vi "example-VariantArrayAccess.vi"() -> ()   [LabVIEW 2020]
uses:
  VariantArrayAccessMulti.vi
panel:
  in  "New Value":cxt
  out "Old Value":variant
  out "Revised Array":variant
  in  "Numeric Array as Variant 2":variant
  out "element":variant
  in  "index":i32
  in  "Array as Variant":variant
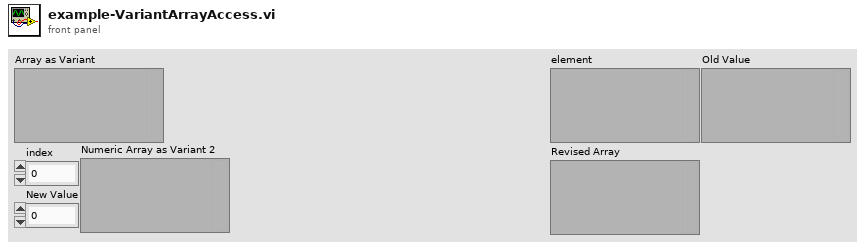
[diagram p1: front panel]
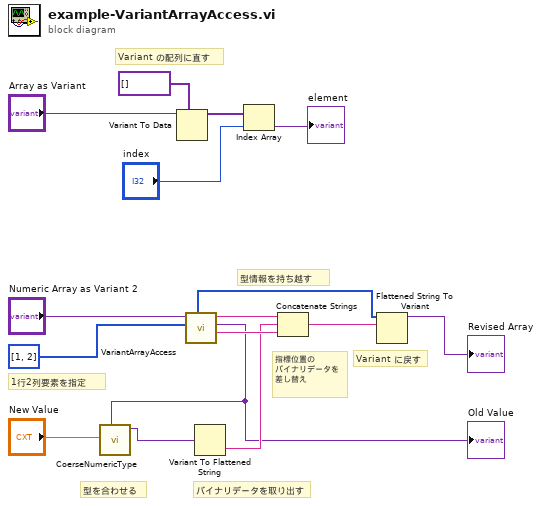
[diagram p0: block diagram]
diagram:
  # "型を合わせる"
  # "Variant に戻す"
  # "型情報を持ち越す"
  # "指標位置の\nバイナリデータを\n差し替え"
  # "バイナリデータを取り出す"
  # "1行2列要素を指定"
  # "Variant の配列に直す"
  n1 = Variant To Data(type=variant[] [], Variant="Array as Variant") -> (data=w15:variant[])  [unwired: 1 in, 1 out]
  n2 = call-poly "VariantArrayAccess.vi"("Indices"=i32[] [1, 2], "Array"="Numeric Array as Variant 2") -> ("rest"=w8:string, "value"=w2:variant, "prepend"=w9:string, "type string"=w6:i16[])  [unwired: 4 in, 2 out]
  "Old Value" <- w2
  n3 = call "CoerseNumericType.vi"("Numeric Variant in"=w2, "Numeric"="New Value") -> ("Numeric Variant out"=w1:variant)  [unwired: 8 in, 1 out]
  n4 = Variant To Flattened String(Variant=w1) -> (data string=w7:string)  [unwired: 1 out]
  n5 = Index Array(array=w15, index="index") -> (element=→"element":variant)
  n6 = Concatenate Strings(w9, w7, w8) -> (w5:string)
  n7 = Flattened String To Variant(6:w5, 7:w6) -> (3:→"Revised Array":variant)  [unwired: 1 in, 1 out]
